vi "plot_rec2circle.vi"(9 "radius":i32, 10 "center of circle":dbl[](array[numeric])) -> (3 "data out":T1)   [LabVIEW 2017]
panel:
  in  "Bounding Rectangle in":T1={"Left"=100, "Top"=100, "Right"=150, "Bottom"=150}
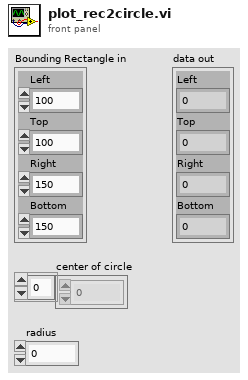
[diagram p1: front panel]
types:
  T1 = cluster{"Left":i32, "Top":i32, "Right":i32, "Bottom":i32}
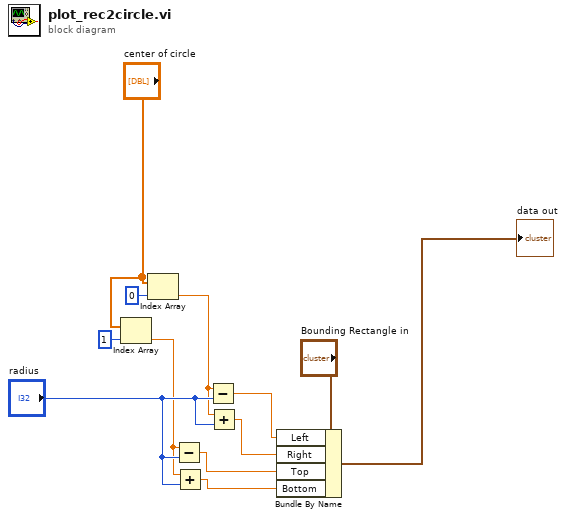
[diagram p0: block diagram]
diagram:
  n1 = Index Array(array="center of circle", index=1) -> (element=w7:dbl)
  n2 = Index Array(array="center of circle", index=0) -> (element=w6:dbl)
  n3 = Subtract(x=w7, y="radius") -> (x-y=w10:dbl)
  n4 = Add(x=w7, y="radius") -> (x+y=w11:dbl)
  n5 = Subtract(x=w6, y="radius") -> (x-y=w5:dbl)
  n6 = Add(x=w6, y="radius") -> (x+y=w9:dbl)
  n7 = Bundle By Name(cluster="Bounding Rectangle in", "Left"=w5, "Right"=w9, "Top"=w10, "Bottom"=w11) -> (→"data out":T1)
